vi "polar.vi"() -> ()   [LabVIEW 2012]
panel:
  in  "stop":bool
  in  "Mag 3":dbl(slide) scale=0.0..10.0
  in  "Phase 3":dbl(knob) scale=0.0..360.0
  in  "Mag 2":dbl(slide) scale=0.0..10.0
  in  "Phase 2":dbl(knob) scale=0.0..360.0
  in  "Mag":dbl(slide) scale=0.0..10.0
  in  "Phase":dbl(knob) scale=0.0..360.0
  out "Polar Plot":picture
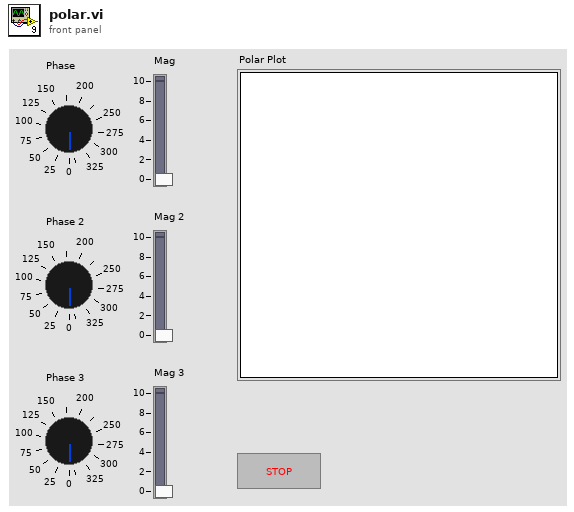
[diagram p1: front panel]
types:
  T1 = cluster{"maximum":dbl, "minimum":dbl, "clip to min":bool, "log?(F)":bool, "grid color":u32, "plot color":u32, "fmt and prec":cluster{"format":enum8{"Decimal", "Scientific", "Engineering", "Binary", "Octal", "Hex"}, "precision":u8}, "visible section":u16}
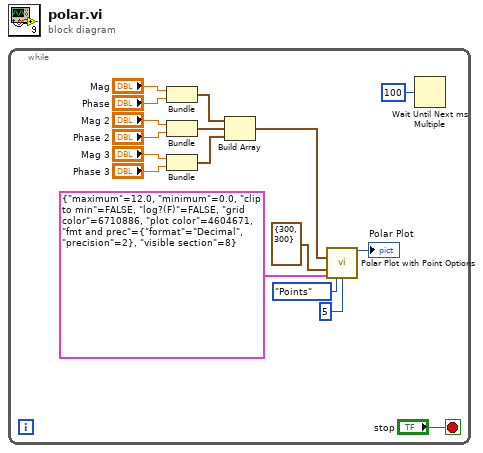
[diagram p0: block diagram]
diagram:
  n1 = while {
    stop <- "stop" stop-if-true
    n2 = Bundle("Mag"="Mag", "Phase"="Phase") -> (w16:cluster{"Mag":dbl, "Phase":dbl})  [unwired: 1 in]
    n3 = Bundle("Mag 2"="Mag 2", "Phase 2"="Phase 2") -> (w17:cluster{"Mag 2":dbl, "Phase 2":dbl})  [unwired: 1 in]
    n4 = Bundle("Mag 3"="Mag 3", "Phase 3"="Phase 3") -> (w15:cluster{"Mag 3":dbl, "Phase 3":dbl})  [unwired: 1 in]
    n5 = Build Array(w16, w17, w15) -> (w14:cluster{"Mag 3":dbl, "Phase 3":dbl}[])
    n6 = call <vilib>:"Polar Plot with Point Options.vi"("data array [mag, phase (deg)]"=w14, "dimensions (w,h)"=cluster{"width":i16, "height":i16} {"width"=300, "height"=300}, "polar attributes"=T1 {"maximum"=12.0, "minimum"=0.0, "clip to min"=FALSE, "log?(F)"=FALSE, "grid color"=6710886, "plot color"=4604671, "fmt and prec"={"format"=enum."Decimal", "precision"=2}, "visible section"=8}, "Lines/Points"=enum16{"Lines", "Points"}."Points", "Size"=u16 5) -> ("new picture"=→"Polar Plot":picture)  [unwired: 10 in]
    n7 = Wait Until Next ms Multiple(millisecond multiple=u32 100) -> ()  [unwired: 1 out]
  }
